vi "SubpanelTemplate.vi"() -> ()   [LabVIEW 2014]
uses:
  Utilities/DataShare/DataShare.lvclass
  Controls/Data.ctl
panel:
  out "Example Generated Data":string[][](table)
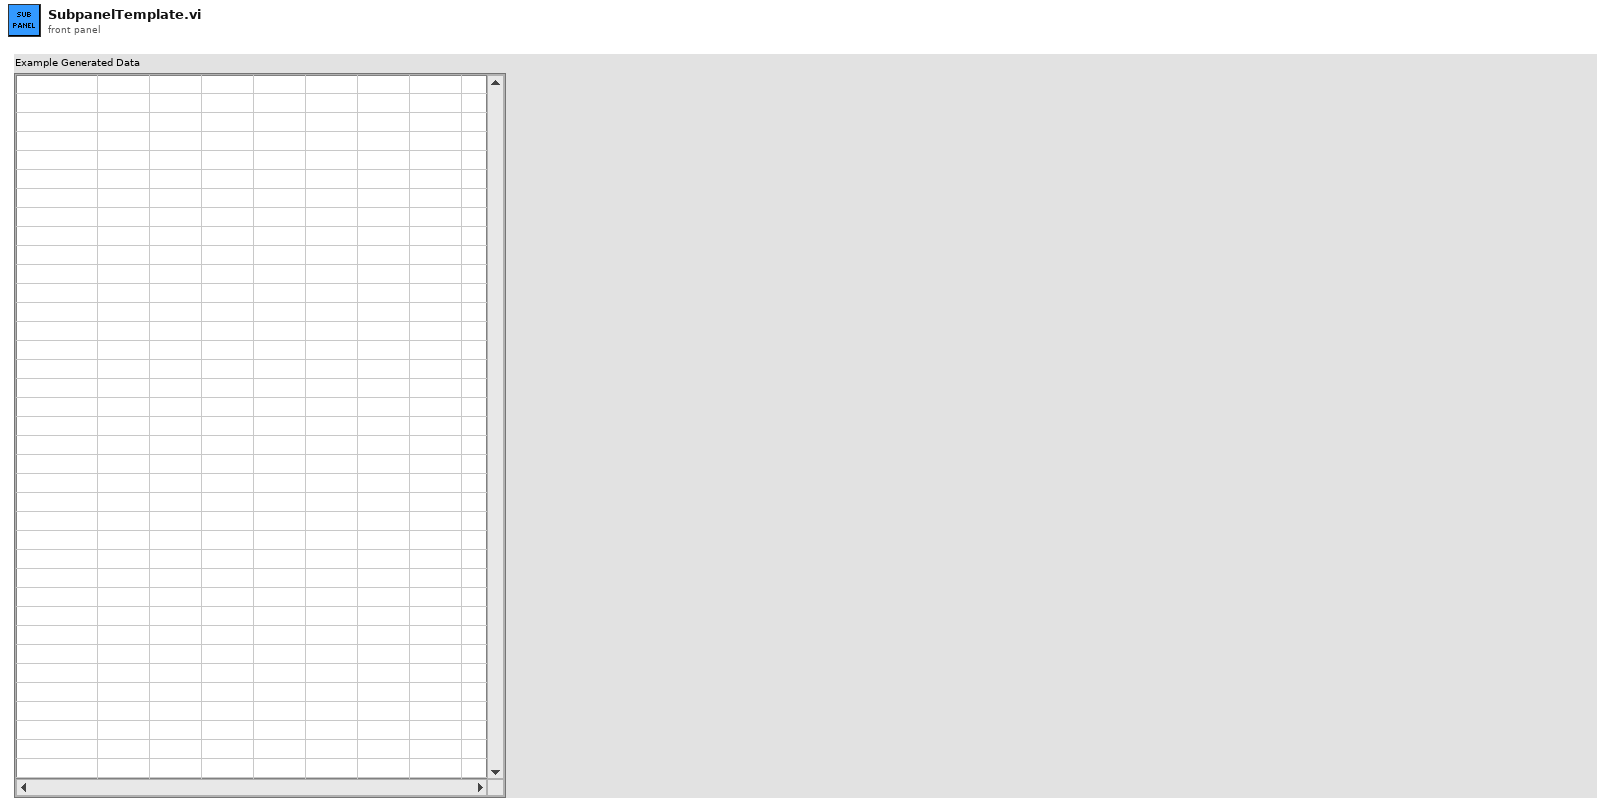
[diagram p1: front panel]
types:
  T1 = typedef "Data.ctl" = cluster{"Names":string[], "Values":dbl[]}
  T2 = cluster{"Error":errorcluster, "Example1":refnum<class "DataShare.lvclass">, "Example2":refnum<class "DataShare.lvclass">, "Data":T1}
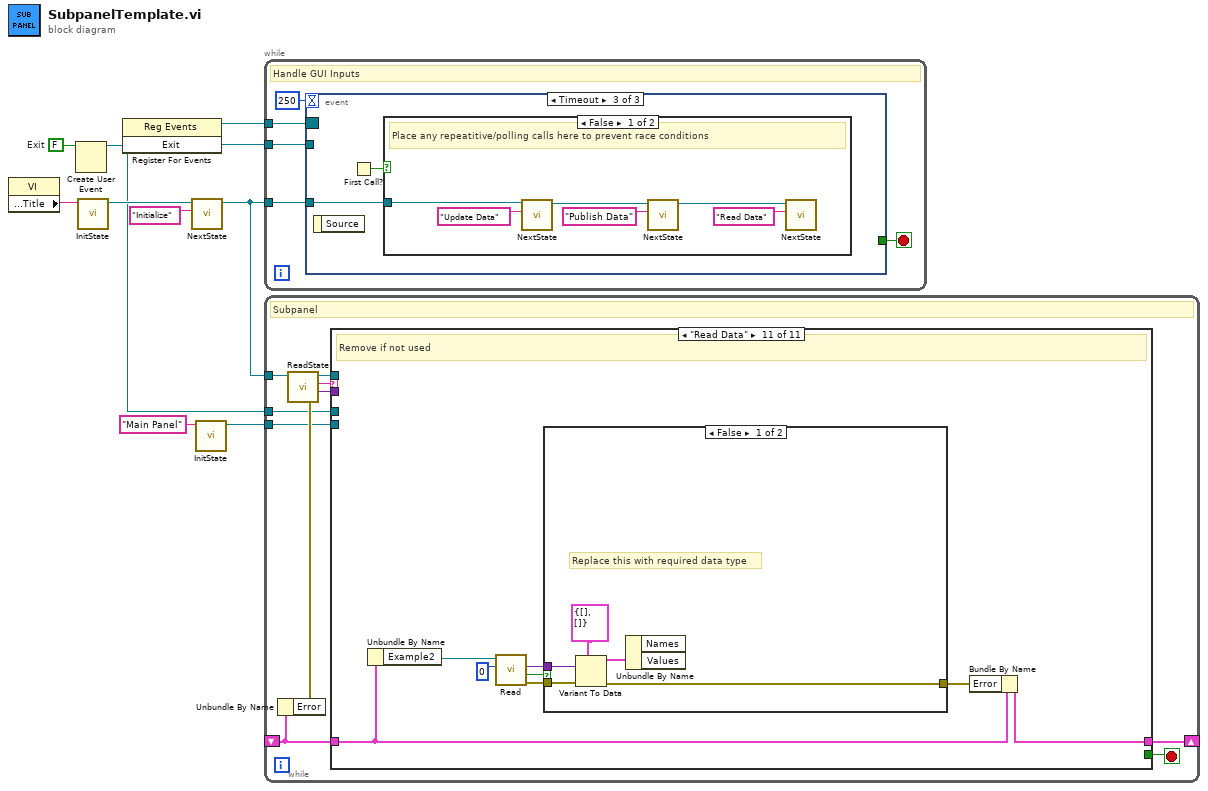
[diagram p0: block diagram]
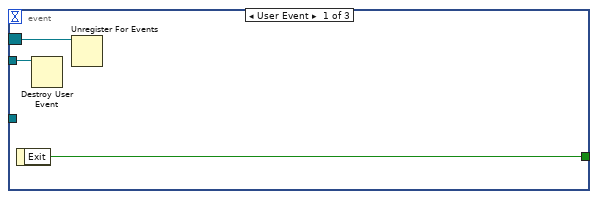
[diagram p2: hidden frame]
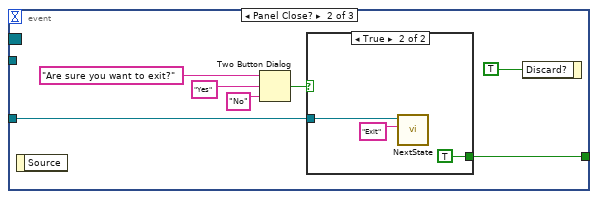
[diagram p3: hidden frame]
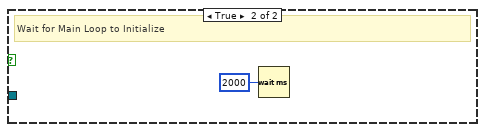
[diagram p5: hidden frame]
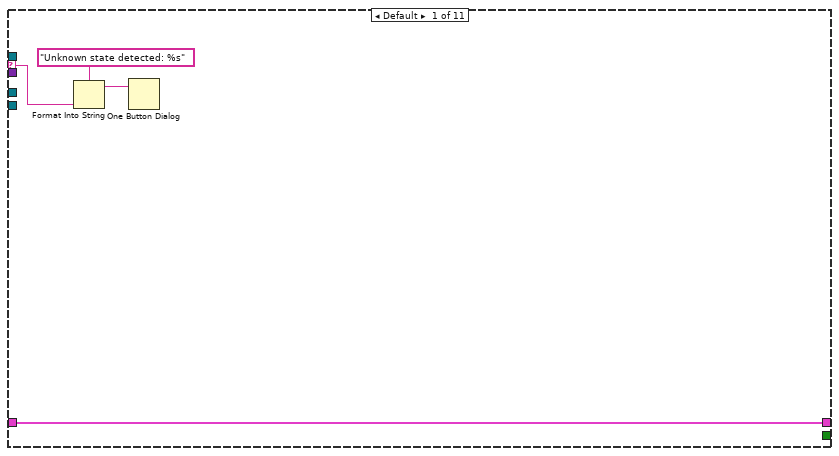
[diagram p6: hidden frame]
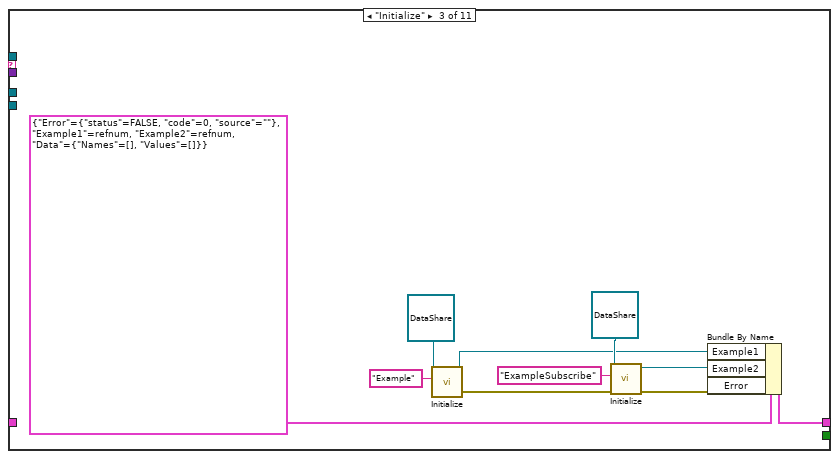
[diagram p8: hidden frame]
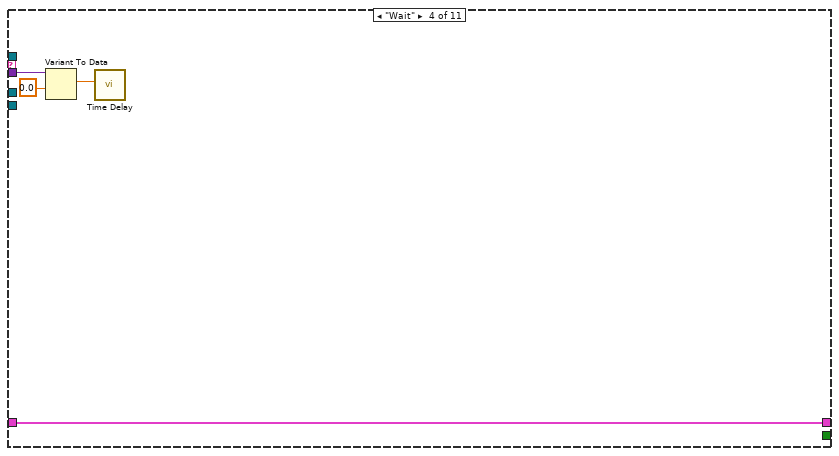
[diagram p9: hidden frame]
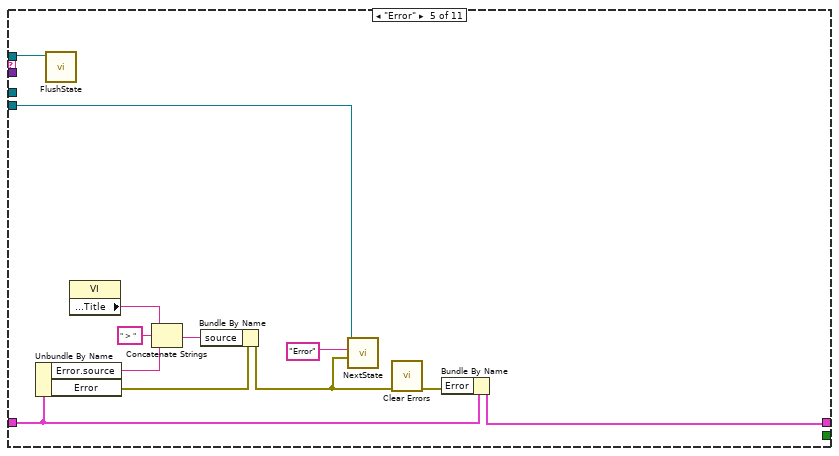
[diagram p10: hidden frame]
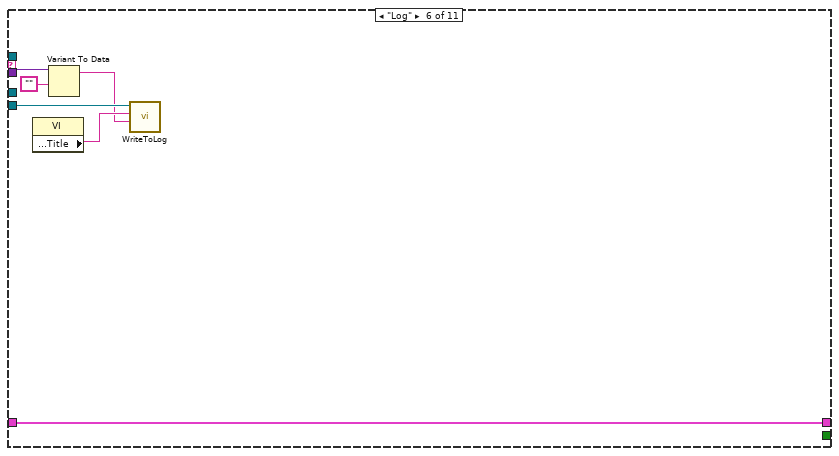
[diagram p11: hidden frame]
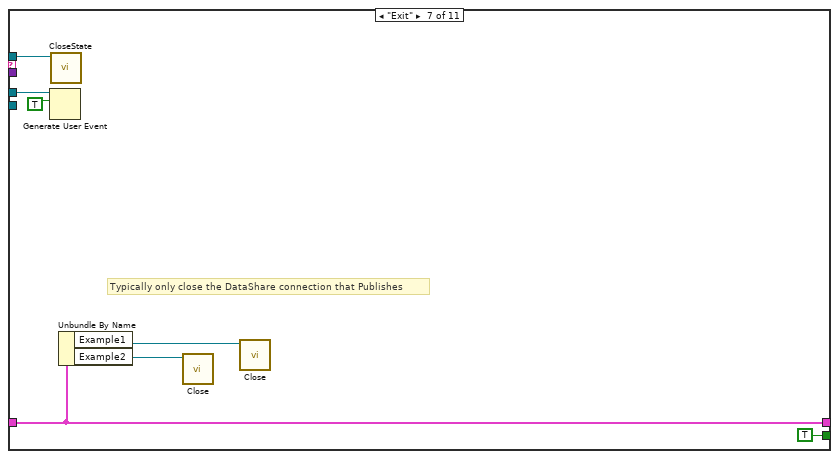
[diagram p12: hidden frame]
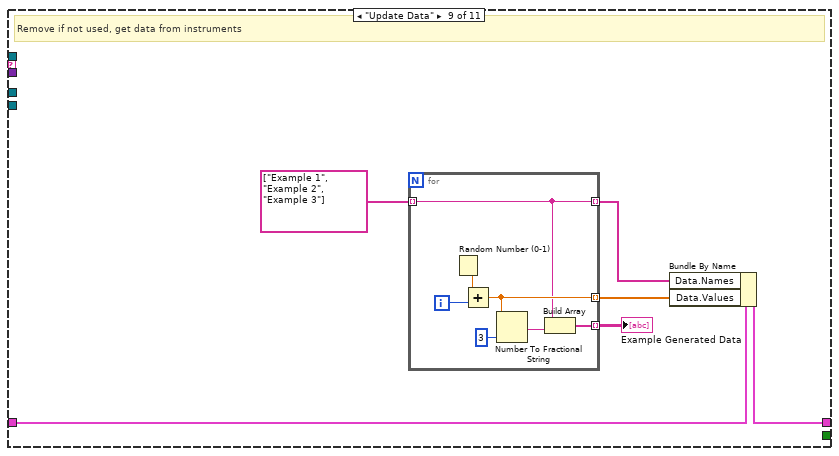
[diagram p14: hidden frame]
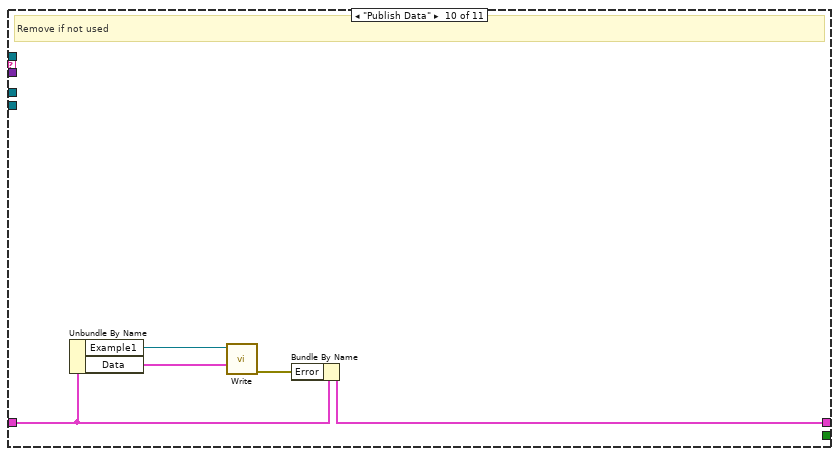
[diagram p15: hidden frame]
diagram:
  w6 = FALSE  # Exit
  n1 = property class="VI"() -> ("Front Panel.Title"=w1:string)  [unwired: 2 in, 2 out]
  n2 = Create User Event(user event datatype=w6) -> (user event=w4:refnum<user-event>)  [unwired: 1 in, 1 out]
  n3 = call "InitState.vi"("Name"=w1) -> ("Queue Out"=w9:refnum<queue>)  [unwired: 8 in, 1 out]
  n4 = register-events(w4) -> (reference out=w5:refnum<event-registration>)  [unwired: 2 in, 1 out]
  n5 = call "NextState.vi"("State"="Initialize" ("element"), "Queue In"=w9) -> ("Queue Out"=w7:refnum<queue>)  [unwired: 8 in, 1 out]
  n6 = call "InitState.vi"("Name"="Main Panel") -> ("Queue Out"=w2:refnum<queue>)  [unwired: 8 in, 1 out]
  n7 = while {
    tunnel: w7 -> [w14]
    tunnel: w5 -> [w12]
    tunnel: w4 -> [w11]
    stop <- w13 stop-if-true
    # "Handle GUI Inputs"
    n8 = event shown="[2] Timeout" {
      selector: w12 -> [w17 _ _]
      dyn-events: _ -> [_ _ _]
      timeout: 250 -> [_ _ _]
      tunnel: w14 -> [_ w19 w29]
      tunnel: [w16 w18 _] -> w13
      tunnel: w11 -> [w15 _ _]
      event User Event {
        n9 = event-data() -> ("Exit"=w16:bool)  [unwired: 1 in]
        n10 = Destroy User Event(user event=w15) -> ()  [unwired: 1 in, 1 out]
        n11 = Unregister For Events(event registration refnum=w17) -> ()  [unwired: 1 in, 1 out]
      }
      event Panel Close? {
        n12 = event-data() -> ()  [unwired: 1 in, 1 out]
        n13 = Two Button Dialog(message="Are sure you want to exit?", 1:"No" ("F button name (\"Cancel\")"), 2:"Yes" ("T button name (\"OK\")")) -> (T button?=w20:bool)
        n14 = case shown="True" w20 {
          tunnel: w19 -> [_ w26]
          tunnel: [_ TRUE] -> w18
          frame False {
          }
          frame True {
            n15 = call "NextState.vi"("State"="Exit" ("element"), "Queue In"=w26) -> ()  [unwired: 8 in, 2 out]
          }
        }
        n16 = event-data("Discard?"=TRUE) -> ()  [unwired: 1 in, 1 out]
      }
      event Timeout {
        n17 = event-data() -> ()  [unwired: 1 in, 1 out]
        n18 = First Call?() -> (First Call?: T/F=w28:bool)
        n19 = case shown="False" w28 {
          tunnel: w29 -> [w31 _]
          frame False {
            # "Place any repeatitive/polling calls here to prevent race conditions"
            n20 = call "NextState.vi"("State"="Update Data" ("element"), "Queue In"=w31) -> ("Queue Out"=w30:refnum<queue>)  [unwired: 8 in, 1 out]
            n21 = call "NextState.vi"("State"="Publish Data" ("element"), "Queue In"=w30) -> ("Queue Out"=w33:refnum<queue>)  [unwired: 8 in, 1 out]
            n22 = call "NextState.vi"("State"="Read Data" ("element"), "Queue In"=w33) -> ()  [unwired: 8 in, 2 out]
          }
          frame True {
            # "Wait for Main Loop to Initialize"
            n23 = Wait (ms)(milliseconds to wait=u32 2000) -> ()  [unwired: 1 out]
          }
        }
      }
    }
  }
  n24 = while {
    tunnel: w7 -> [w44]
    shift-right: [w46] -> _
    shift-left: _ -> [w40]
    tunnel: w4 -> [w38]
    tunnel: w2 -> [w37]
    stop <- w45 stop-if-true
    # "Subpanel"
    n25 = Unbundle By Name(w40) -> ("Error"=w39:errorcluster)
    n26 = call "ReadState.vi"("Error In"=w39, "Queue In"=w44) -> ("Data"=w41:variant, "State"=w42:string, "Queue Out"=w43:refnum<queue>)  [unwired: 6 in, 1 out]
    n27 = case shown="\"Read Data\"" w42 {
      tunnel: w41 -> [_ _ _ w65 _ w82 _ _ _ _ _]
      selector: w42 -> [w49 _ _ _ _ _ _ _ _ _ _]
      tunnel: [w47 w51 w56 w62 w77 w79 w86 w91 w93 w107 w110] -> w46
      tunnel: [_ _ _ _ _ _ TRUE _ _ _ _] -> w45
      tunnel: w40 -> [w47 w51 _ w62 w76 w79 w86 w91 w94 w108 w113]
      tunnel: w43 -> [_ _ _ _ w75 _ w87 _ _ _ _]
      tunnel: w38 -> [_ _ _ _ _ _ w89 _ _ _ _]
      tunnel: w37 -> [_ _ _ _ w74 w83 _ _ _ _ _]
      frame Default {
        n28 = Format Into String(format string="Unknown state detected: %s", w49) -> (resulting string=w48:string)  [unwired: 2 in, 1 out]
        n29 = One Button Dialog(message=w48) -> ()  [unwired: 1 in, 1 out]
      }
      frame "--- System ---" {
      }
      frame "Initialize" {
        n30 = call "Initialize.vi"("Name"="Example", "DataShare in"=refnum<class "DataShare.lvclass"> refnum) -> ("error out"=w52:errorcluster, "DataShare out"=w53:refnum<class "DataShare.lvclass">)  [unwired: 8 in]
        n31 = call "Initialize.vi"("error in (no error)"=w52, "Name"="ExampleSubscribe", "DataShare in"=refnum<class "DataShare.lvclass"> refnum) -> ("error out"=w55:errorcluster, "DataShare out"=w54:refnum<class "DataShare.lvclass">)  [unwired: 7 in]
        n32 = Bundle By Name(cluster=T2 {"Error"={"status"=FALSE, "code"=0, "source"=""}, "Example1"=refnum, "Example2"=refnum, "Data"={"Names"=[], "Values"=[]}}, "Example1"=w53, "Example2"=w54, "Error"=w55) -> (w56:T2)
      }
      frame "Wait" {
        n33 = Variant To Data(type=0.0, Variant=w65) -> (data=w63:dbl)  [unwired: 1 in, 1 out]
        n34 = call "Time Delay"("Delay Time (s)"=w63) -> ()  [unwired: 10 in, 1 out]
      }
      frame "Error" {
        n35 = Unbundle By Name(w76) -> ("Error.source"=w67:string, "Error"=w71:errorcluster)
        n36 = call "FlushState.vi"("Queue In"=w75) -> ()  [unwired: 9 in, 2 out]
        n37 = property class="VI"() -> ("Front Panel.Title"=w68:string)  [unwired: 2 in, 2 out]
        n38 = Concatenate Strings(w68, " > " ("string"), w67) -> (w66:string)
        n39 = Bundle By Name(cluster=w71, "source"=w66) -> (w70:errorcluster)
        n40 = call "NextState.vi"("Data"=w70, "State"="Error", "Queue In"=w74) -> ()  [unwired: 7 in, 2 out]
        n41 = call <vilib>:"Clear Errors.vi"("error in (no error)"=w70) -> ("error out"=w72:errorcluster)  [unwired: 5 in, 1 out]
        n42 = Bundle By Name(cluster=w76, "Error"=w72) -> (w77:T2)
      }
      frame "Log" {
        n43 = property class="VI"() -> ("Front Panel.Title"=w81:string)  [unwired: 2 in, 2 out]
        n44 = Variant To Data(type="", Variant=w82) -> (data=w80:string)  [unwired: 1 in, 1 out]
        n45 = call "WriteToLog.vi"("Data"=w80, "Source"=w81, "Queue In"=w83) -> ()  [unwired: 7 in, 2 out]
      }
      frame "Exit" {
        # "Typically only close the DataShare connection that Publishes"
        n46 = Generate User Event(user event=w89, event data cluster=TRUE ("event data")) -> ()  [unwired: 2 in, 2 out]
        n47 = call "CloseState.vi"("Queue In"=w87) -> ()  [unwired: 10 in, 1 out]
        n48 = Unbundle By Name(w86) -> ("Example1"=w84:refnum<class "DataShare.lvclass">, "Example2"=w85:refnum<class "DataShare.lvclass">)
        n49 = call "Close.vi"("DataShare in"=w85) -> ()  [unwired: 9 in, 2 out]
        n50 = call "Close.vi"("DataShare in"=w84) -> ()  [unwired: 9 in, 2 out]
      }
      frame "--- Customize This ---" {
      }
      frame "Update Data" {
        # "Remove if not used, get data from instruments"
        n51 = for {
          tunnel: string[] ["Example 1", "Example 2", "Example 3"] -> [w99] mode=indexing
          tunnel: [w99] -> w95 mode=indexing
          tunnel: [w102] -> w96 mode=indexing
          tunnel: [w98] -> w92 mode=indexing
          i -> [w103]
          n52 = Random Number (0-1)() -> (number: 0 to 1=w104:dbl)
          n53 = Add(x=w104, y=w103) -> (x+y=w102:dbl)
          n54 = Number To Fractional String(number=w102, precision (6)=i16 3) -> (F-format string=w100:string)  [unwired: 2 in]
          n55 = Build Array(w99, w100) -> (w98:string[])
        }
        "Example Generated Data" <- w92
        n56 = Bundle By Name(cluster=w94, "Data.Names"=w95, "Data.Values"=w96) -> (w93:T2)
      }
      frame "Publish Data" {
        # "Remove if not used"
        n57 = Unbundle By Name(w108) -> ("Example1"=w109:refnum<class "DataShare.lvclass">, "Data"=w105:T1)
        n58 = call "Write.vi"("Data"=w105, "DataShare in"=w109) -> ("error out"=w106:errorcluster)  [unwired: 8 in, 1 out]
        n59 = Bundle By Name(cluster=w108, "Error"=w106) -> (w107:T2)
      }
      frame "Read Data" {
        # "Remove if not used"
        n60 = Unbundle By Name(w113) -> ("Example2"=w117:refnum<class "DataShare.lvclass">)
        n61 = call "Read.vi"("Timeout"=0, "DataShare in"=w117) -> ("error out"=w112:errorcluster, "Timed Out?"=w115:bool, "Data"=w114:variant)  [unwired: 6 in, 1 out]
        n62 = case shown="False" w115 {
          tunnel: w114 -> [w122 _]
          tunnel: w112 -> [w119 w123]
          tunnel: [w118 w123] -> w111
          frame False {
            # "Replace this with required data type"
            n63 = Variant To Data(error in=w119, type=T1 {"Names"=[], "Values"=[]} ("Data"), Variant=w122) -> (data=w120:T1, error out=w118:errorcluster)
            n64 = Unbundle By Name(w120) -> ()  [unwired: 2 out]
          }
          frame True {
          }
        }
        n65 = Bundle By Name(cluster=w113, "Error"=w111) -> (w110:T2)
      }
    }
  }
